vi "File.Source Path to Dest Path, relative to Source Root Folder.vi"(7 "Dest Folder":path, 10 "Root Path":path, 11 "File Path":path) -> (2 "SubDirCnt":i32, 3 "Dest Path":path)   [LabVIEW 2018]
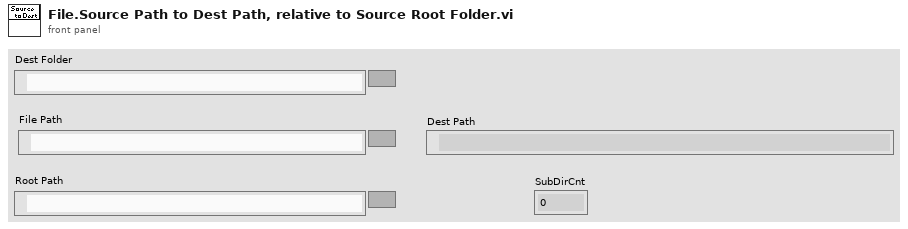
[diagram p1: front panel]
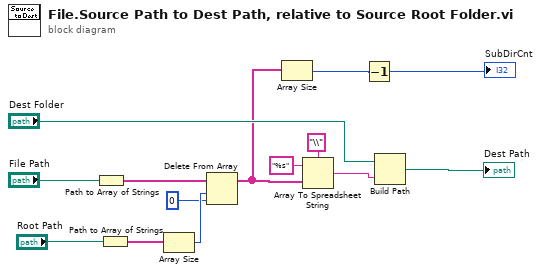
[diagram p0: block diagram]
diagram:
  n1 = Path to Array of Strings(0:"File Path") -> (2:w11:string[])  [unwired: 1 out]
  n2 = Path to Array of Strings(0:"Root Path") -> (2:w12:string[])  [unwired: 1 out]
  n3 = Array Size(array=w12) -> (size(s)=w10:i32)
  n4 = Delete From Array(array=w11, length=w10, index=0) -> (array with subset deleted=w3:string[])  [unwired: 1 out]
  n5 = Array Size(array=w3) -> (size(s)=w2:i32)
  n6 = Array To Spreadsheet String(delimiter (Tab)="\\", array=w3, 3:"%s" ("format string")) -> (spreadsheet string=w4:string)
  n7 = Decrement(x=w2) -> (x-1=→"SubDirCnt":i32)
  n8 = Build Path(base path="Dest Folder", name or relative path=w4) -> (appended path=→"Dest Path":path)
